vi "distance_formula.vi"(1 "X2 - X1":dbl, 2 "Y2 - Y1":dbl) -> (0 "Distance":dbl)   [LabVIEW 2011]
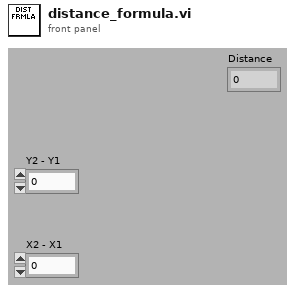
[diagram p1: front panel]
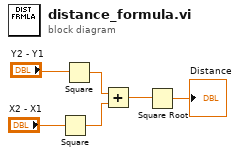
[diagram p0: block diagram]
diagram:
  n1 = Square(x="X2 - X1") -> (x^2=w3:dbl)
  n2 = Square(x="Y2 - Y1") -> (x^2=w4:dbl)
  n3 = Add(x=w4, y=w3) -> (x+y=w2:dbl)
  n4 = Square Root(x=w2) -> (sqrt(x)=→"Distance":dbl)
